vi "CIA main.vi"(6 "init":bool) -> ()   [LabVIEW 2018]
uses:
  CIA_IRQ_oper.ctl
  CIA1_glb.vi
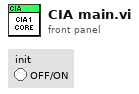
[diagram p1: front panel]
types:
  T1 = typedef "CIA_IRQ_oper.ctl" = enum16{"init", "set mask", "set flag", "check active", "read reg"}
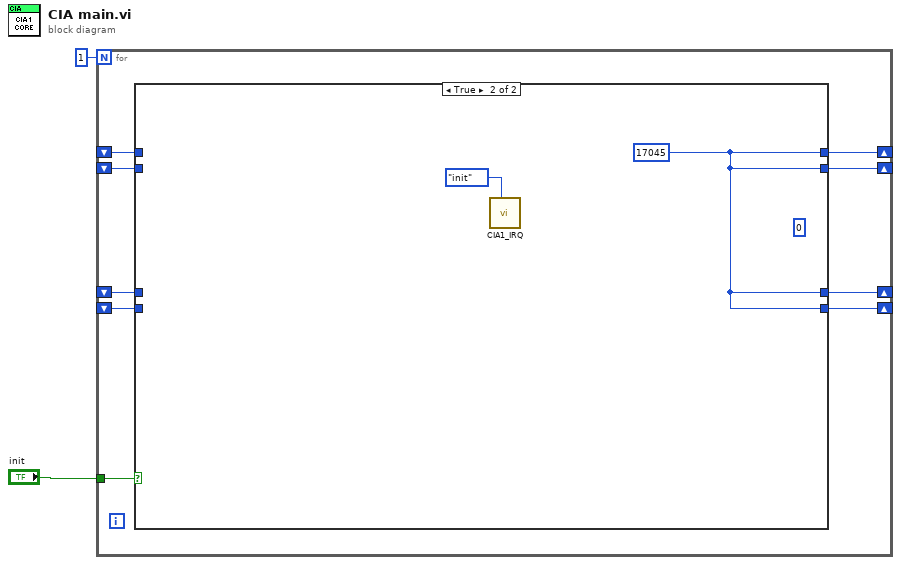
[diagram p0: block diagram]
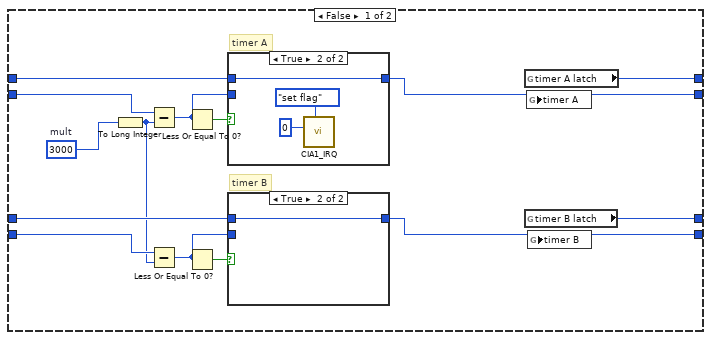
[diagram p2: hidden frame]
diagram:
  n1 = for {
    N: 1 -> [_]
    shift-right: [w11] -> _
    shift-left: _ -> [w10]
    tunnel: "init" -> [w9]
    shift-right: [w8] -> _
    shift-left: _ -> [w7]
    shift-right: [w3] -> _
    shift-left: _ -> [w4]
    shift-right: [w5] -> _
    shift-left: _ -> [w6]
    n2 = case shown="True" w9 {
      tunnel: [w22 w32] -> w11
      tunnel: w10 -> [w25 _]
      tunnel: [w23 w32] -> w8
      tunnel: w7 -> [w24 _]
      tunnel: [w21 w32] -> w3
      tunnel: w4 -> [w18 _]
      tunnel: [w20 w32] -> w5
      tunnel: w6 -> [w19 _]
      frame False {
        w12 = u32 3000  # mult
        # "timer A"
        # "timer B"
        n3 = To Long Integer(number=w12) -> (32bit integer=w13:i32)
        n4 = Subtract(x=w25, y=w13) -> (x-y=w17:i32)
        n5 = Subtract(x=w18, y=w13) -> (x-y=w14:i32)
        n6 = Less Or Equal To 0?(x=w17) -> (x <= 0?=w16:bool)
        n7 = Less Or Equal To 0?(x=w14) -> (x <= 0?=w15:bool)
        n8 = case shown="True" w16 {
          tunnel: w24 -> [_ w31]
          tunnel: [w28 w31] -> w22
          tunnel: w17 -> [w28 _]
          frame False {
          }
          frame True {
            n9 = call "CIA1_IRQ.vi"("oper"=CIA_IRQ_oper."set flag", "IRQ flag idx"=u8 0) -> ()  [unwired: 8 in, 2 out]
          }
        }
        n10 = case shown="True" w15 {
          tunnel: w19 -> [_ w27]
          tunnel: [w26 w27] -> w21
          tunnel: w14 -> [w26 _]
          frame False {
          }
          frame True {
          }
        }
        n11 = global read "CIA1_glb.vi" "timer A latch"() -> (w23:i32)
        n12 = global read "CIA1_glb.vi" "timer B latch"() -> (w20:i32)
        n13 = global write "CIA1_glb.vi" "timer A"(w22) -> ()
        n14 = global write "CIA1_glb.vi" "timer B"(w21) -> ()
      }
      frame True {
        (unwired) u16 0
        w32 = u16 17045
        n15 = call "CIA1_IRQ.vi"("oper"=CIA_IRQ_oper."init") -> ()  [unwired: 9 in, 2 out]
      }
    }
  }
